vi "计算中高频Z.vi"(0 "特性阻抗Z0":dbl, 2 "r":cdb[](array[numeric]), 5 "x3":dbl, 7 "factor":dbl, 9 "L":dbl, 11 "H43":cdb[](array[numeric]), 12 "k":cdb[](array[numeric])) -> (4 "Z中高频":cdb[](array[numeric]))   [LabVIEW 2018]
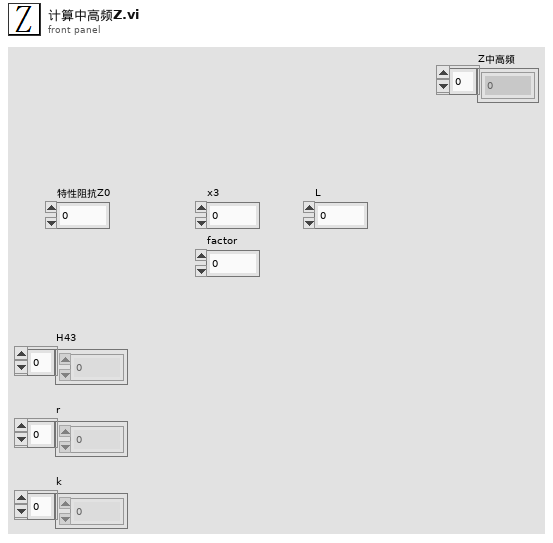
[diagram p1: front panel]
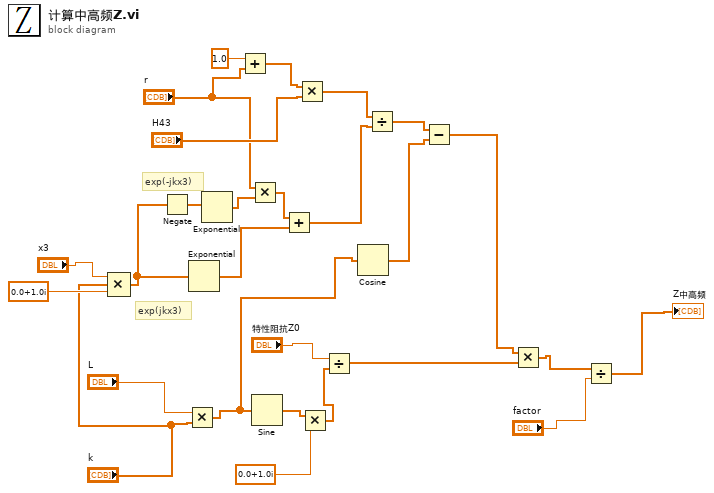
[diagram p0: block diagram]
diagram:
  # "exp(jkx3)"
  # "exp(-jkx3)"
  n1 = Compound Arithmetic op=MULTIPLY("x3", "k", cdb 0.0+1.0i) -> (w11:cdb[])
  n2 = Negate(x=w11) -> (-x=w10:cdb[])
  n3 = Multiply(x="L", y="k") -> (x*y=w5:cdb[])
  n4 = Exponential(1:w11) -> (0:w12:cdb[])
  n5 = Exponential(1:w10) -> (0:w9:cdb[])
  n6 = Add(x=1.0, y="r") -> (x+y=w18:cdb[])
  n7 = Multiply(x="r", y=w9) -> (x*y=w7:cdb[])
  n8 = Sine(x=w5) -> (sin(x)=w25:cdb[])
  n9 = Add(x=w7, y=w12) -> (x+y=w6:cdb[])
  n10 = Multiply(x=w18, y="H43") -> (x*y=w21:cdb[])
  n11 = Multiply(x=w25, y=cdb 0.0+1.0i) -> (x*y=w23:cdb[])
  n12 = Divide(x="特性阻抗Z0", y=w23) -> (x/y=w22:cdb[])
  n13 = Cosine(x=w5) -> (cos(x)=w4:cdb[])
  n14 = Divide(x=w21, y=w6) -> (x/y=w20:cdb[])
  n15 = Subtract(x=w20, y=w4) -> (x-y=w19:cdb[])
  n16 = Multiply(x=w19, y=w22) -> (x*y=w3:cdb[])
  n17 = Divide(x=w3, y="factor") -> (x/y=→"Z中高频":cdb[])
